vi "Header Licor-Data.vi"(7 "Licor-Sources":T1[](array[typedef])) -> (8 "Header":string[](array[string]))   [LabVIEW 2010]
uses:
  Licor-Steuerung/LicorLI7000/conventions/Licor-Source.ctl
  Licor-Steuerung/LicorLI7000/LicorLI7000.lvlib
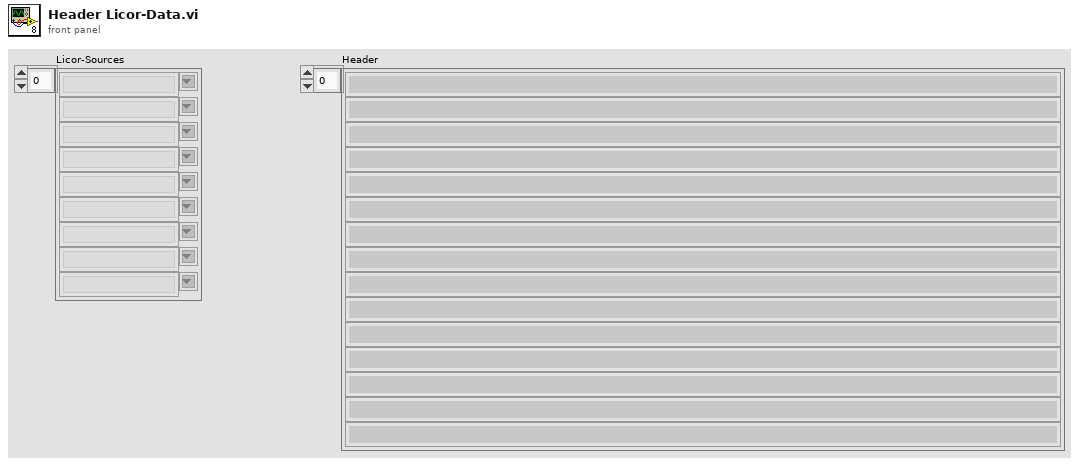
[diagram p1: front panel]
types:
  T1 = typedef "LicorLI7000.lvlib/Licor-Source.ctl" = string
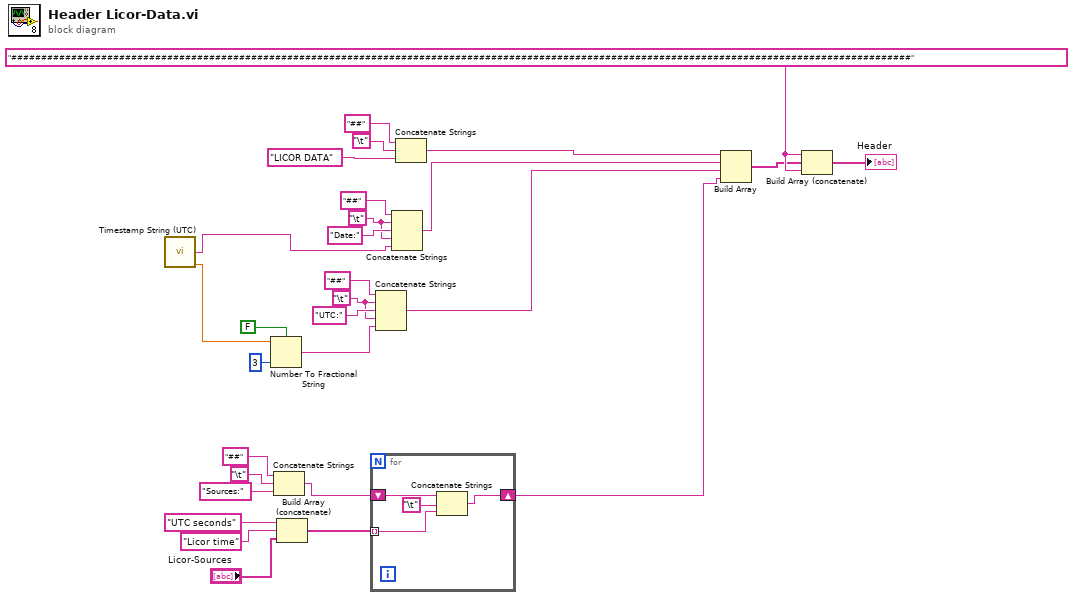
[diagram p0: block diagram]
diagram:
  w11 = "\t"
  w15 = "\t"
  w29 = "######################################################################################################################################################"
  n1 = call "Timestamp String (UTC).vi"() -> ("date/time string (UTC)"=w6:string, "UTC [s]"=w5:dbl)  [unwired: 14 in]
  n2 = Number To Fractional String(use system decimal point (T)=FALSE ("Systemdezimalzeichen verwenden (T)"), number=w5, precision (6)=i16 3 ("Genauigkeit (6)")) -> (F-format string=w9:string)  [unwired: 1 in]
  n3 = Concatenate Strings("##", "\t", "Sources:") -> (w23:string)
  n4 = Build Array (concatenate)("UTC seconds" ("group name"), "Licor time" ("group name"), "Licor-Sources") -> (w2:T1[])
  n5 = for {
    tunnel: w2 -> [w31] mode=indexing
    shift-right: [w30] -> w14
    shift-left: w23 -> [w33]
    n6 = Concatenate Strings(w33, "\t", w31) -> (w30:string)
  }
  n7 = Concatenate Strings("##", w11, "UTC:" ("String"), w11, w9) -> (w8:string)
  n8 = Concatenate Strings("##", w15, "Date:" ("String"), w15, w6) -> (w17:string)
  n9 = Concatenate Strings("##", "\t", "LICOR DATA") -> (w19:string)
  n10 = Build Array(w19, w17, w8, w14) -> (w28:string[])
  n11 = Build Array (concatenate)(w29, w28, w29) -> (→"Header":string[])
